vi "get_pv_dimensions.vi"(10 "stream_handle":u64, 11 "path in":path=path "hl2ss_ulm.dll") -> (0 "height":u16, 1 "width":u16, 2 "stream_handle":u64, 3 "path out":path, 4 "error":bool)   [LabVIEW 2023]
panel:
  in  "height":u16
  in  "width":u16
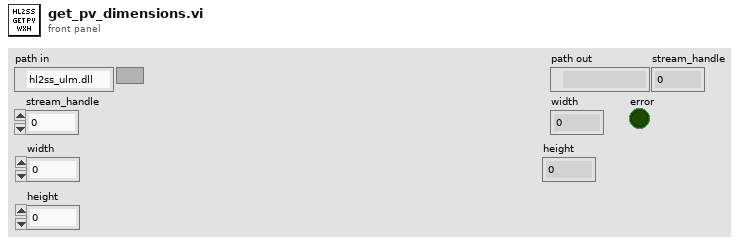
[diagram p1: front panel]
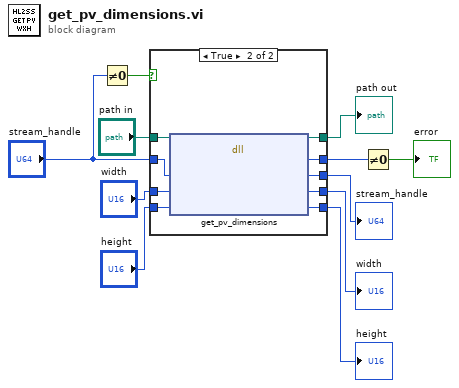
[diagram p0: block diagram]
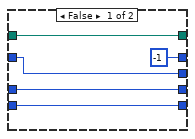
[diagram p2: hidden frame]
diagram:
  n1 = Not Equal To 0?(x="stream_handle") -> (x != 0?=w11:bool)
  n2 = case shown="True" w11 {
    tunnel: "path in" -> [w15 w25]
    tunnel: "stream_handle" -> [w16 w24]
    tunnel: [w15 w23] -> w9
    tunnel: [w16 w22] -> w8
    tunnel: "width" -> [w13 w21]
    tunnel: "height" -> [w12 w20]
    tunnel: [-1 ("return type") w19] -> w3
    tunnel: [w13 w18] -> w2
    tunnel: [w12 w17] -> w1
    frame False {
    }
    frame True {
      n3 = dll-call lib="C:/Users/jcds/Documents/GitHub/hl2ss/extensions/client_labview/hl2ss_labview/hl2ss_ulm.dll" fn="get_pv_dimensions"(path in=w25, "handle"=w24, "width"=w21, "height"=w20) -> (path out=w23:path, "return type"=w19:i32, "handle"=w22:u64, "width"=w18:u16, "height"=w17:u16)  [unwired: 2 in, 1 out]
    }
  }
  "path out" <- w9
  "stream_handle" <- w8
  "width" <- w2
  "height" <- w1
  n4 = Not Equal To 0?(x=w3) -> (x != 0?=→"error":bool)
